vi "General_Setup_string.vi"() -> (0 "Output string":string)   [LabVIEW 2010]
uses:
  Controls/Graph_Type.ctl
  Globals/Preference_global.vi
  Globals/Meas_global.vi
  Globals/Trav_pos_global.vi
panel:
  in  "Plot Type":T1=enum."Voltage trace"
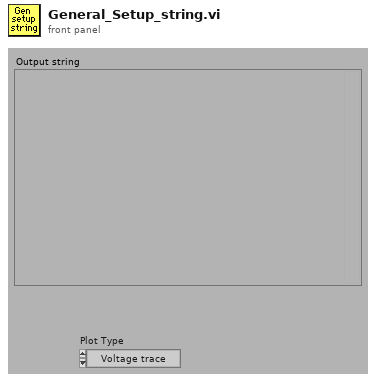
[diagram p1: front panel]
types:
  T1 = typedef "Graph_Type.ctl" = enum16{"Show no graph", "Voltage trace", "Velocity trace", "Vel histogram", "Spectrum", "f.E(f) v Log f", "Auto-Corr"}
  T2 = typedef "Board_Types.ctl" = enum16{"Simulate", "Local ADAM", "Server ADAM", "NI-DAQmx", "NI-DAQmxBase", "ADC488", "DT LV-link"}
  T3 = enum16{"From String to Cluster", "From Cluster to String"}
  T4 = cluster{"Plot 1":u16, "Plot 2":u16, "Save graph":u16, "Plot Type":T1}
  T5 = enum16{"Save no data", "Save data in new files", "Save data in existing files"}
  T6 = typedef "Tunnel_Coordinates.ctl" = enum16{"Work in Tunnel Coordinates", "Work in Model Coordinates"}
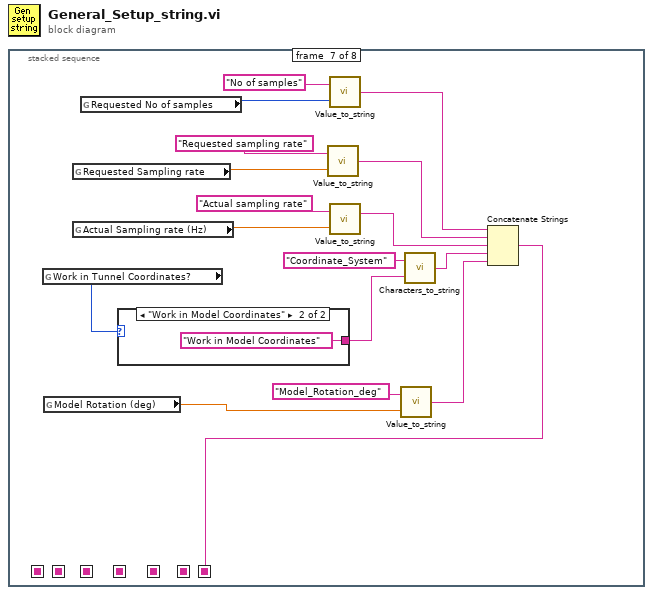
[diagram p0: block diagram]
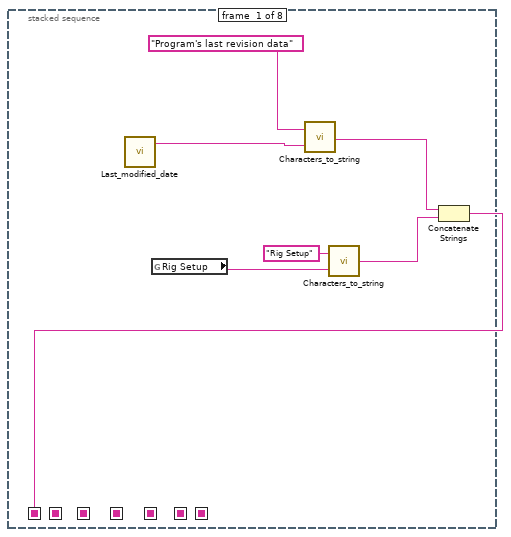
[diagram p2: hidden frame]
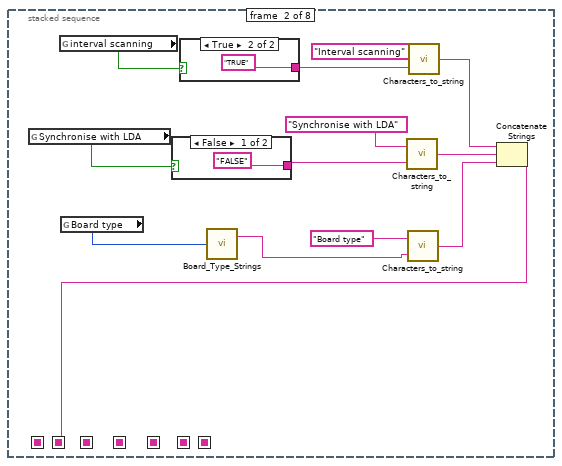
[diagram p3: hidden frame]
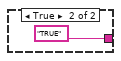
[diagram p4: hidden frame]
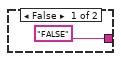
[diagram p5: hidden frame]
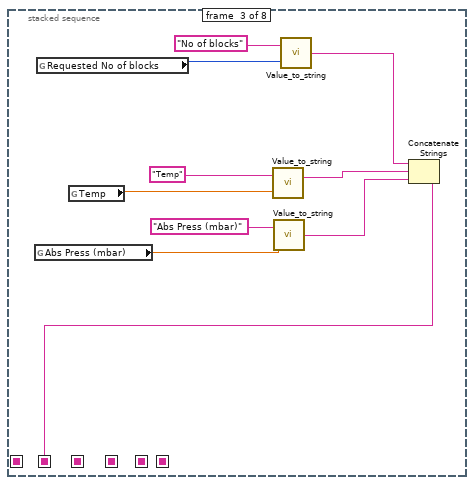
[diagram p6: hidden frame]
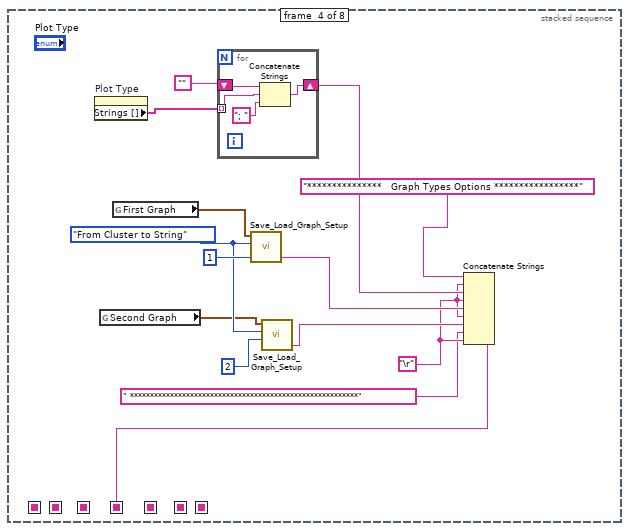
[diagram p7: hidden frame]
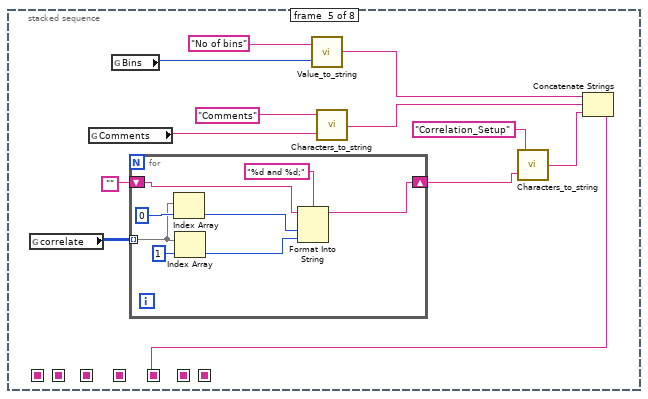
[diagram p8: hidden frame]
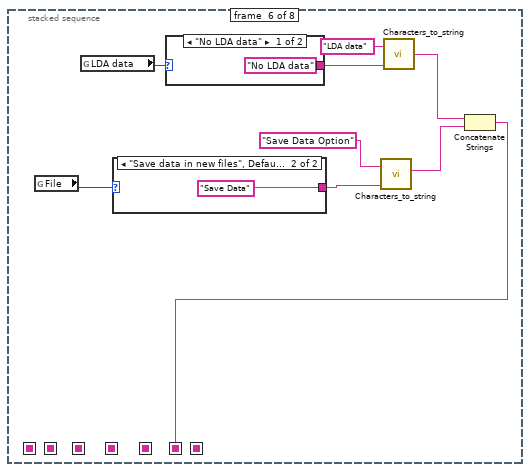
[diagram p9: hidden frame]
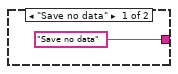
[diagram p10: hidden frame]
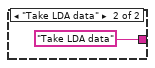
[diagram p11: hidden frame]
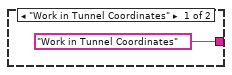
[diagram p12: hidden frame]
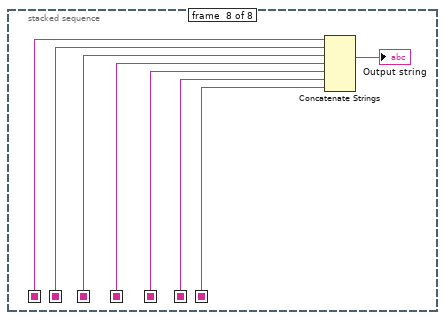
[diagram p13: hidden frame]
diagram:
  n1 = stacked-sequence {
    seq-local: [_ _ w32 _ _ _ _ _] -> [_ _ _ _ _ _ _ w112]
    seq-local: [_ w14 _ _ _ _ _ _] -> [_ _ _ _ _ _ _ w111]
    seq-local: [_ _ _ _ _ w73 _ _] -> [_ _ _ _ _ _ _ w107]
    seq-local: [_ _ _ _ _ _ w98 _] -> [_ _ _ _ _ _ _ w106]
    seq-local: [_ _ _ w48 _ _ _ _] -> [_ _ _ _ _ _ _ w109]
    seq-local: [_ _ _ _ w59 _ _ _] -> [_ _ _ _ _ _ _ w108]
    seq-local: [w7 _ _ _ _ _ _ _] -> [_ _ _ _ _ _ _ w105]
    frame #0 {
      n2 = call "Last_modified_date.vi"() -> ("Output string"=w2:string)  [unwired: 1 in, 1 out]
      n3 = global read "Preference_global.vi" "Rig Setup"() -> (w4:string)
      n4 = call "Characters_to_string.vi"("Characters to write"=w2, "Label for characters"="Program's last revision data") -> ("Output string"=w1:string)
      n5 = call "Characters_to_string.vi"("Characters to write"=w4, "Label for characters"="Rig Setup") -> ("Output string"=w5:string)
      n6 = Concatenate Strings(w1, w5) -> (w7:string)
    }
    frame #1 {
      n7 = global read "Meas_global.vi" "Synchronise with LDA"() -> (w11:bool)
      n8 = global read "Meas_global.vi" "interval scanning"() -> (w13:bool)
      n9 = global read "Meas_global.vi" "Board type"() -> (w9:T2)
      n10 = case shown="False" w11 {
        tunnel: ["FALSE" "TRUE"] -> w10
        frame False {
        }
        frame True {
        }
      }
      n11 = case shown="True" w13 {
        tunnel: ["FALSE" "TRUE"] -> w12
        frame False {
        }
        frame True {
        }
      }
      n12 = call "Board_Type_Strings.vi"("Board type"=w9) -> ("Board String"=w8:string)  [unwired: 1 out]
      n13 = call "Characters_to_string.vi"("Characters to write"=w10, "Label for characters"="Synchronise with LDA") -> ("Output string"=w16:string)
      n14 = call "Characters_to_string.vi"("Characters to write"=w8, "Label for characters"="Board type") -> ("Output string"=w15:string)
      n15 = call "Characters_to_string.vi"("Characters to write"=w12, "Label for characters"="Interval scanning") -> ("Output string"=w17:string)
      n16 = Concatenate Strings(w17, w16, w15) -> (w14:string)
    }
    frame #2 {
      n17 = global read "Meas_global.vi" "Abs Press (mbar)"() -> (w29:dbl)
      n18 = global read "Meas_global.vi" "Requested No of blocks"() -> (w33:i32)
      n19 = global read "Meas_global.vi" "Temp"() -> (w28:dbl)
      n20 = call "Value_to_string.vi"("Value"=w28, "Label for value"="Temp") -> ("Output string"=w27:string)  [unwired: 1 in]
      n21 = call "Value_to_string.vi"("Value"=w29, "Label for value"="Abs Press (mbar)") -> ("Output string"=w26:string)  [unwired: 1 in]
      n22 = call "Value_to_string.vi"("Value"=w33, "Label for value"="No of blocks") -> ("Output string"=w25:string)  [unwired: 1 in]
      n23 = Concatenate Strings(w25, w27, w26) -> (w32:string)
    }
    frame #3 {
      w38 = "\r"
      w45 = T3."From Cluster to String" ("Mode")
      n24 = property on="Plot Type" class="Enum (strict)"() -> ("Strings []"=w40:string[])  [unwired: 2 in, 2 out]
      n25 = global read "Meas_global.vi" "Second Graph"() -> (w44:T4)
      n26 = global read "Meas_global.vi" "First Graph"() -> (w41:T4)
      n27 = for {
        shift-right: [w51] -> w39
        shift-left: "" -> [w52]
        tunnel: w40 -> [w50] mode=indexing
        n28 = Concatenate Strings(w52, w50, "; " ("string")) -> (w51:string)
      }
      n29 = call "Save_Load_Graph_Setup.vi"("Graph Number"=1, "Mode"=w45, "Graph in"=w41) -> ("Setup String Out"=w42:string)  [unwired: 1 in, 2 out]
      n30 = call "Save_Load_Graph_Setup.vi"("Graph Number"=2, "Mode"=w45, "Graph in"=w44) -> ("Setup String Out"=w43:string)  [unwired: 1 in, 2 out]
      n31 = Concatenate Strings("***************   Graph Types Options *****************", w38, w39, w38, w42, w38, w43, " *********************************************************" ("string"), w38) -> (w48:string)
    }
    frame #4 {
      n32 = global read "Meas_global.vi" "correlate"() -> (w57:i32[][])
      n33 = global read "Meas_global.vi" "Comments"() -> (w58:string)
      n34 = global read "Meas_global.vi" "Bins"() -> (w63:i32)
      n35 = for {
        tunnel: w57 -> [w70] mode=indexing
        shift-right: [w66] -> w54
        shift-left: "" -> [w67]
        n36 = Index Array(array=w70, index=0) -> (element=w69:i32)
        n37 = Index Array(array=w70, index=1) -> (element=w68:i32)
        n38 = Format Into String(format string="%d and %d;", initial string=w67, w69, w68) -> (resulting string=w66:string)  [unwired: 1 in, 1 out]
      }
      n39 = call "Value_to_string.vi"("Value"=w63, "Label for value"="No of bins") -> ("Output string"=w62:string)  [unwired: 1 in]
      n40 = call "Characters_to_string.vi"("Characters to write"=w58, "Label for characters"="Comments") -> ("Output string"=w60:string)
      n41 = call "Characters_to_string.vi"("Characters to write"=w54, "Label for characters"="Correlation_Setup") -> ("Output string"=w53:string)
      n42 = Concatenate Strings(w62, w60, w53) -> (w59:string)
    }
    frame #5 {
      n43 = global read "Meas_global.vi" "File"() -> (w78:T5)
      n44 = global read "Meas_global.vi" "LDA data"() -> (w79:enum16{"No LDA data", "Take LDA data"})
      n45 = case shown="\"Save data in new files\", Default" w78 {
        tunnel: ["Save no data" "Save Data"] -> w76
        frame "Save no data" {
        }
        frame "Save data in new files", Default {
        }
      }
      n46 = case shown="\"No LDA data\"" w79 {
        tunnel: ["No LDA data" "Take LDA data"] -> w80
        frame "No LDA data" {
        }
        frame "Take LDA data" {
        }
      }
      n47 = call "Characters_to_string.vi"("Characters to write"=w76, "Label for characters"="Save Data Option") -> ("Output string"=w74:string)
      n48 = call "Characters_to_string.vi"("Characters to write"=w80, "Label for characters"="LDA data") -> ("Output string"=w75:string)
      n49 = Concatenate Strings(w75, w74) -> (w73:string)
    }
    frame #6 {
      n50 = global read "Trav_pos_global.vi" "Work in Tunnel Coordinates?"() -> (w95:T6)
      n51 = global read "Trav_pos_global.vi" "Model Rotation (deg)"() -> (w90:dbl)
      n52 = global read "Meas_global.vi" "Requested Sampling rate"() -> (w88:dbl)
      n53 = global read "Meas_global.vi" "Actual Sampling rate (Hz)"() -> (w99:dbl)
      n54 = global read "Meas_global.vi" "Requested No of samples"() -> (w101:i32)
      n55 = case shown="\"Work in Model Coordinates\"" w95 {
        tunnel: ["Work in Tunnel Coordinates" "Work in Model Coordinates"] -> w94
        frame "Work in Tunnel Coordinates" {
        }
        frame "Work in Model Coordinates" {
        }
      }
      n56 = call "Value_to_string.vi"("Value"=w88, "Label for value"="Requested sampling rate") -> ("Output string"=w86:string)  [unwired: 1 in]
      n57 = call "Value_to_string.vi"("Value"=w101, "Label for value"="No of samples") -> ("Output string"=w97:string)  [unwired: 1 in]
      n58 = call "Value_to_string.vi"("Value"=w99, "Label for value"="Actual sampling rate") -> ("Output string"=w96:string)  [unwired: 1 in]
      n59 = call "Value_to_string.vi"("Value"=w90, "Label for value"="Model_Rotation_deg" ("Label for characters")) -> ("Output string"=w89:string)  [unwired: 1 in]
      n60 = call "Characters_to_string.vi"("Characters to write"=w94, "Label for characters"="Coordinate_System") -> ("Output string"=w92:string)
      n61 = Concatenate Strings(w97, w86, w96, w92, w89) -> (w98:string)
    }
    frame #7 {
      n62 = Concatenate Strings(w105, w111, w112, w109, w108, w107, w106) -> (→"Output string":string)
    }
  }
